vi "CTRE_PigeonIMU_GetData.vi"   [LabVIEW 2016]
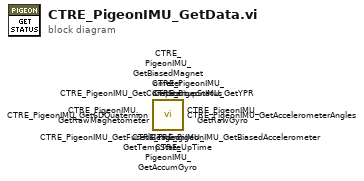
[diagram p0: block diagram]
diagram:
  n1 = call <vilib>:"CTRE_PigeonIMU_GetTempStateUpTime.vi"() -> ()  [unwired: 9 in, 3 out]
  n2 = call <vilib>:"CTRE_PigeonIMU_GetStartupStatus.vi"() -> ()  [unwired: 9 in, 3 out]
  n3 = call <vilib>:"CTRE_PigeonIMU_GetRawMagnetometer.vi"() -> ()  [unwired: 9 in, 3 out]
  n4 = call <vilib>:"CTRE_PigeonIMU_GetRawGyro.vi"() -> ()  [unwired: 9 in, 3 out]
  n5 = call <vilib>:"CTRE_PigeonIMU_GetCompass.vi"() -> ()  [unwired: 9 in, 3 out]
  n6 = call <vilib>:"CTRE_PigeonIMU_GetBiasedMagnetometer.vi"() -> ()  [unwired: 9 in, 3 out]
  n7 = call <vilib>:"CTRE_PigeonIMU_GetBiasedAccelerometer.vi"() -> ()  [unwired: 9 in, 3 out]
  n8 = call <vilib>:"CTRE_PigeonIMU_GetAccumGyro.vi"() -> ()  [unwired: 9 in, 3 out]
  n9 = call <vilib>:"CTRE_PigeonIMU_GetAccelerometerAngles.vi"() -> ()  [unwired: 9 in, 3 out]
  n10 = call <vilib>:"CTRE_PigeonIMU_Get6DQuaternion.vi"() -> ()  [unwired: 9 in, 3 out]
  n11 = call <vilib>:"CTRE_PigeonIMU_GetFusedHeading.vi"() -> ()  [unwired: 9 in, 3 out]
  n12 = call <vilib>:"CTRE_PigeonIMU_GetYPR.vi"() -> ()  [unwired: 9 in, 3 out]
